vi "voorliggerdetectie.vi"() -> ()   [LabVIEW 2019]
panel:
  out "linkerwiel":dbl(knob) scale=0.0..10.0
  in  "linkerwiel":dbl(slide) scale=0.0..10.0
  in  "stop":bool
  in  "voorliggerdetectie":bool
  out "rechterwiel":dbl(knob) scale=0.0..10.0
  in  "rechterwiel":dbl(slide) scale=0.0..10.0
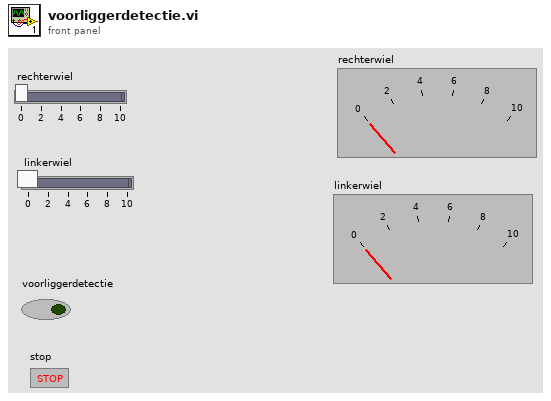
[diagram p1: front panel]
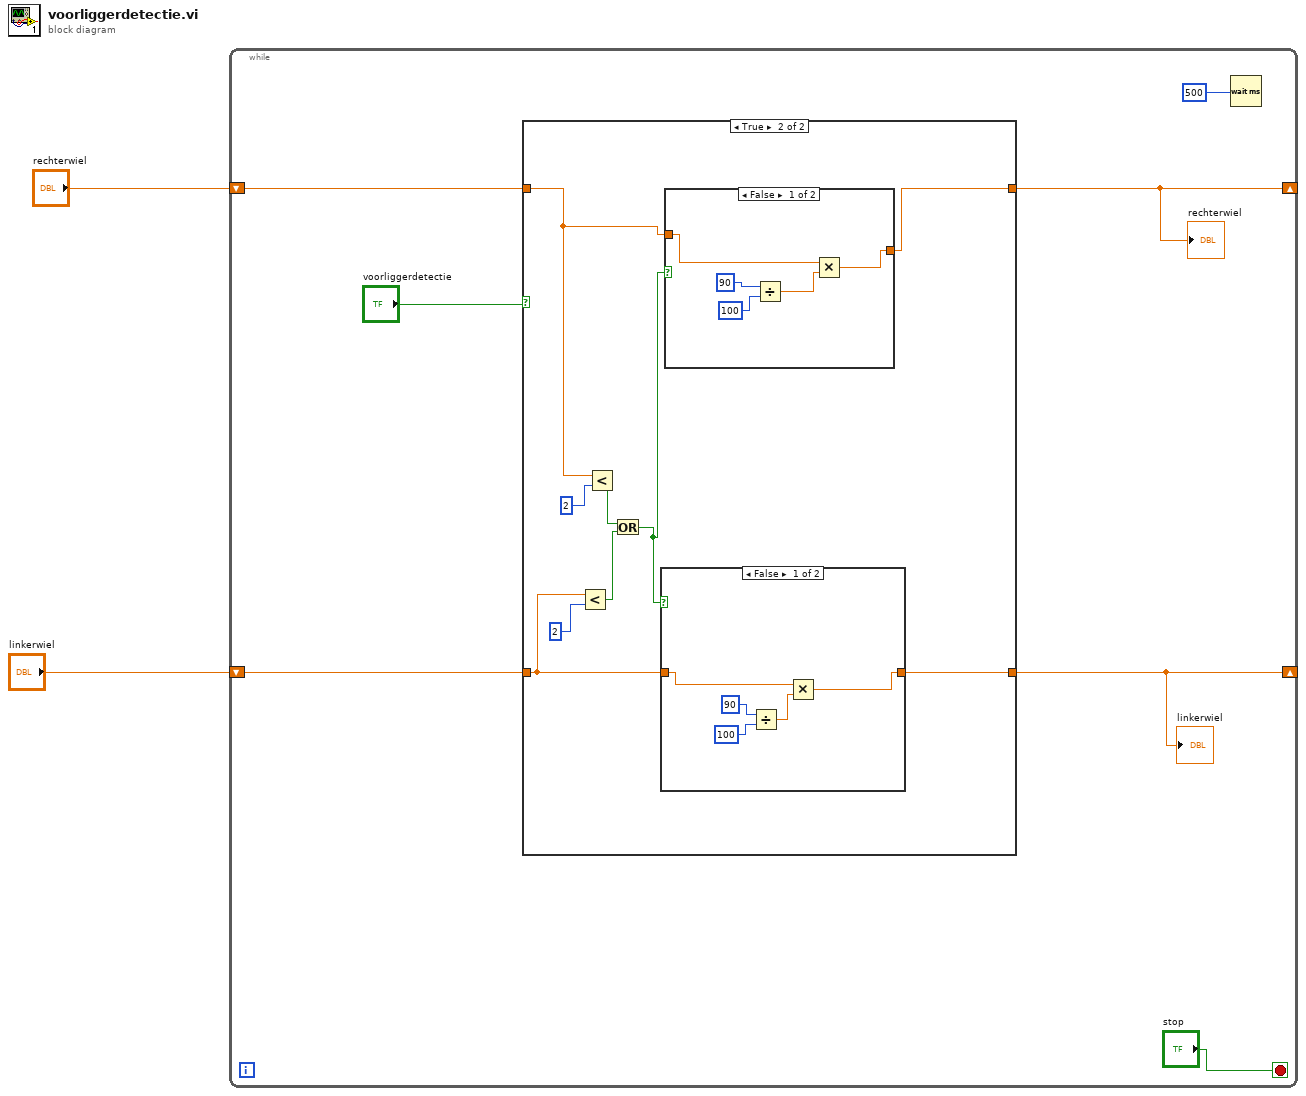
[diagram p0: block diagram]
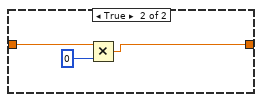
[diagram p3: hidden frame]
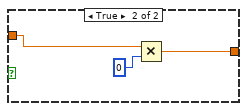
[diagram p4: hidden frame]
diagram:
  n1 = while {
    shift-right: [w7] -> _
    shift-left: "rechterwiel" -> [w9]
    shift-right: [w3] -> _
    shift-left: "linkerwiel" -> [w4]
    stop <- "stop" stop-if-true
    n2 = case shown="True" "voorliggerdetectie" {
      tunnel: w9 -> [w11 w19]
      tunnel: [w11 w18] -> w7
      tunnel: w4 -> [w10 w16]
      tunnel: [w10 w15] -> w3
      frame False {
      }
      frame True {
        n3 = Less?(x=w16, y=2) -> (x < y?=w13:bool)
        n4 = Less?(x=w19, y=2) -> (x < y?=w14:bool)
        n5 = Or(x=w14, y=w13) -> (x .or. y?=w12:bool)
        n6 = case shown="False" w12 {
          tunnel: w16 -> [w22 w28]
          tunnel: [w21 w27] -> w15
          frame False {
            n7 = Divide(x=90, y=100) -> (x/y=w23:dbl)
            n8 = Multiply(x=w22, y=w23) -> (x*y=w21:dbl)
          }
          frame True {
            n9 = Multiply(x=w28, y=0) -> (x*y=w27:dbl)
          }
        }
        n10 = case shown="False" w12 {
          tunnel: w19 -> [w30 w35]
          tunnel: [w29 w34] -> w18
          frame False {
            n11 = Divide(x=90, y=100) -> (x/y=w31:dbl)
            n12 = Multiply(x=w30, y=w31) -> (x*y=w29:dbl)
          }
          frame True {
            n13 = Multiply(x=w35, y=0) -> (x*y=w34:dbl)
          }
        }
      }
    }
    "rechterwiel" <- w7
    "linkerwiel" <- w3
    n14 = Wait (ms)(milliseconds to wait=500) -> ()  [unwired: 1 out]
  }
